vi "SortPics.vi"() -> ()   [LabVIEW 2014]
uses:
  <userlib>/Nanonis Prog Interface V5/Nanonis Prog Interface.lvlib
panel:
  in  "deco":bool
  in  "skip":bool
  out "name":string
  out "new path":path
  in  "unstable":bool
  in  "LowRes":bool
  in  "Multiple":bool
  in  "Good":bool
  in  "method":T1(ring)
  out "Img1":picture
  in  "Read channel 2":i8 min=-1
  in  "Path":path=path "D:/STM Data/082016/160823_095600_2mol_chain/topo"
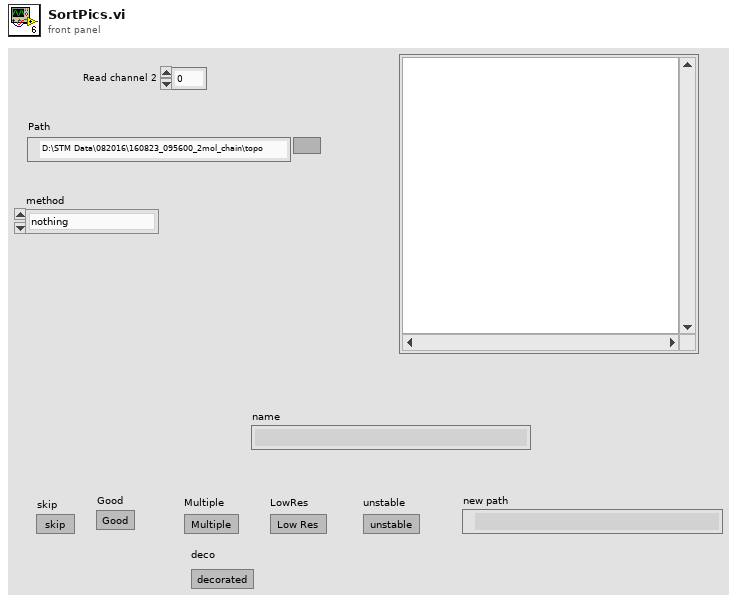
[diagram p1: front panel]
types:
  T1 = enum16{"nothing", "average", "8bit", "average/plane", "minimum", "plane", "average/stddev", "plane/average"}
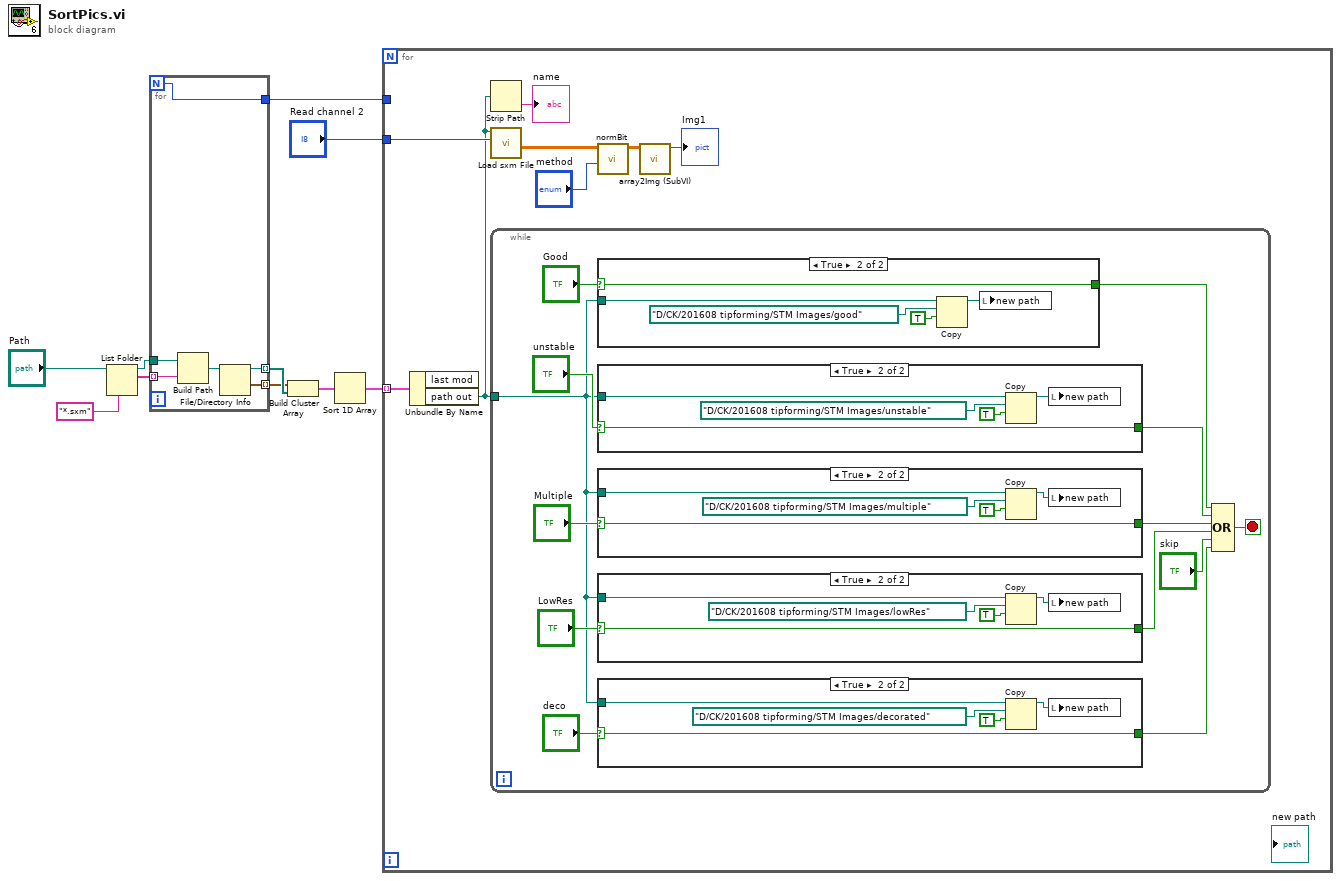
[diagram p0: block diagram]
diagram:
  n1 = List Folder(path="Path", pattern="*.sxm") -> (path out=w7:path, filenames=w8:string[])  [unwired: 2 in, 2 out]
  n2 = for {
    N -> [w11]
    tunnel: w8 -> [w16] mode=indexing
    tunnel: w7 -> [w15]
    tunnel: [w13] -> w4 mode=indexing
    tunnel: [w12] -> w5 mode=indexing
    tunnel: [w11] -> w1
    n3 = Build Path(base path=w15, name or relative path=w16) -> (appended path=w14:path)
    n4 = File/Directory Info(path=w14) -> (path out=w12:path, last mod=w13:timestamp)  [unwired: 1 in, 5 out]
  }
  n5 = Build Cluster Array(w4, w5) -> (w3:cluster{"last mod":timestamp, "path out":path}[])
  n6 = Sort 1D Array(array=w3) -> (sorted array=w2:cluster{"last mod":timestamp, "path out":path}[])
  n7 = for {
    tunnel: "Read channel 2" -> [w24]
    tunnel: w2 -> [w20] mode=indexing
    tunnel: w1 -> [_]
    n8 = Unbundle By Name(w20) -> ("path out"=w18:path)  [unwired: 1 out]
    n9 = Strip Path(path=w18) -> (name=→"name":string)  [unwired: 1 out]
    n10 = call <userlib>:"Load sxm File.vi"("Read channel"=w24, "Scan data file"=w18) -> ("Data"=w22:sgl[][])  [unwired: 4 in, 5 out]
    n11 = while {
      tunnel: w18 -> [w26]
      stop <- w32 stop-if-true
      n12 = case shown="True" "Good" {
        selector: "Good" -> [w62 w64]
        tunnel: w26 -> [_ w67]
        tunnel: [w62 w64] -> w33
        frame False {
        }
        frame True {
          n13 = Copy(9:TRUE ("overwrite (F)"), 10:path "D:/CK/201608 tipforming/STM Images/good" ("target path (use dialog)"), 11:w67) -> (3:w65:path)  [unwired: 2 in, 2 out]
          n14 = local write "new path"(w65) -> ()
        }
      }
      n15 = case shown="True" "unstable" {
        selector: "unstable" -> [w44 w46]
        tunnel: w26 -> [_ w49]
        tunnel: [w44 w46] -> w31
        frame False {
        }
        frame True {
          n16 = Copy(9:TRUE ("overwrite (F)"), 10:path "D:/CK/201608 tipforming/STM Images/unstable" ("target path (use dialog)"), 11:w49) -> (3:w47:path)  [unwired: 2 in, 2 out]
          n17 = local write "new path"(w47) -> ()
        }
      }
      n18 = case shown="True" "Multiple" {
        selector: "Multiple" -> [w56 w58]
        tunnel: w26 -> [_ w61]
        tunnel: [w56 w58] -> w30
        frame False {
        }
        frame True {
          n19 = Copy(9:TRUE ("overwrite (F)"), 10:path "D:/CK/201608 tipforming/STM Images/multiple" ("target path (use dialog)"), 11:w61) -> (3:w59:path)  [unwired: 2 in, 2 out]
          n20 = local write "new path"(w59) -> ()
        }
      }
      n21 = case shown="True" "LowRes" {
        selector: "LowRes" -> [w50 w52]
        tunnel: w26 -> [_ w55]
        tunnel: [w50 w52] -> w29
        frame False {
        }
        frame True {
          n22 = Copy(9:TRUE ("overwrite (F)"), 10:path "D:/CK/201608 tipforming/STM Images/lowRes" ("target path (use dialog)"), 11:w55) -> (3:w53:path)  [unwired: 2 in, 2 out]
          n23 = local write "new path"(w53) -> ()
        }
      }
      n24 = case shown="True" "deco" {
        selector: "deco" -> [w38 w40]
        tunnel: w26 -> [_ w43]
        tunnel: [w38 w40] -> w27
        frame False {
        }
        frame True {
          n25 = Copy(9:TRUE ("overwrite (F)"), 10:path "D:/CK/201608 tipforming/STM Images/decorated" ("target path (use dialog)"), 11:w43) -> (3:w41:path)  [unwired: 2 in, 2 out]
          n26 = local write "new path"(w41) -> ()
        }
      }
      n27 = Compound Arithmetic op=OR(w33, w31, w30, w29, "skip", w27) -> (w32:bool)
    }
    n28 = call "normBit.vi"("method"="method", "Rxy"=w22) -> ("Array"=w19:dbl[][])  [unwired: 8 in, 1 out]
    n29 = call "array2Img (SubVI).vi"("Rxy"=w19) -> ("new picture"=→"Img1":picture)  [unwired: 10 in]
  }
